vi "particle.vi"() -> ()   [LabVIEW 2017]
panel:
  in  "Strength":i32=1
  in  "Power law":i32=2
  in  "Cursor":enum16{"Attract", "Repel", "No interaction"}(ring)
  in  "Trail length":i32=500
  in  "millisecond timer value":u32=2
  in  "Drag":dbl(knob)=0.6535267495370096 scale=0.0..10.0
  in  "G":dbl[](array[numeric])=[0.0, 0.0]
  in  "Initial Velocity":dbl[](array[numeric])=[10.0, 10.0]
  in  "Initial Position":dbl[](array[numeric])=[30.0, 50.0]
  in  "?":bool
  out "XY Graph":cluster{dbl[], dbl[]}[](graph)=[{[58.5077894120906], [41.27386237710225]}, {array[500 elements], array[500 elements]}, {[46.86915887850467, 56.86915887850467, 56.86915887850467, 46.86915887850467, 46.86915887850467], [39.529262086513995, 39.529262086513995, 49.529262086513995, 49.529262086513995, 39.529262086513995]}]
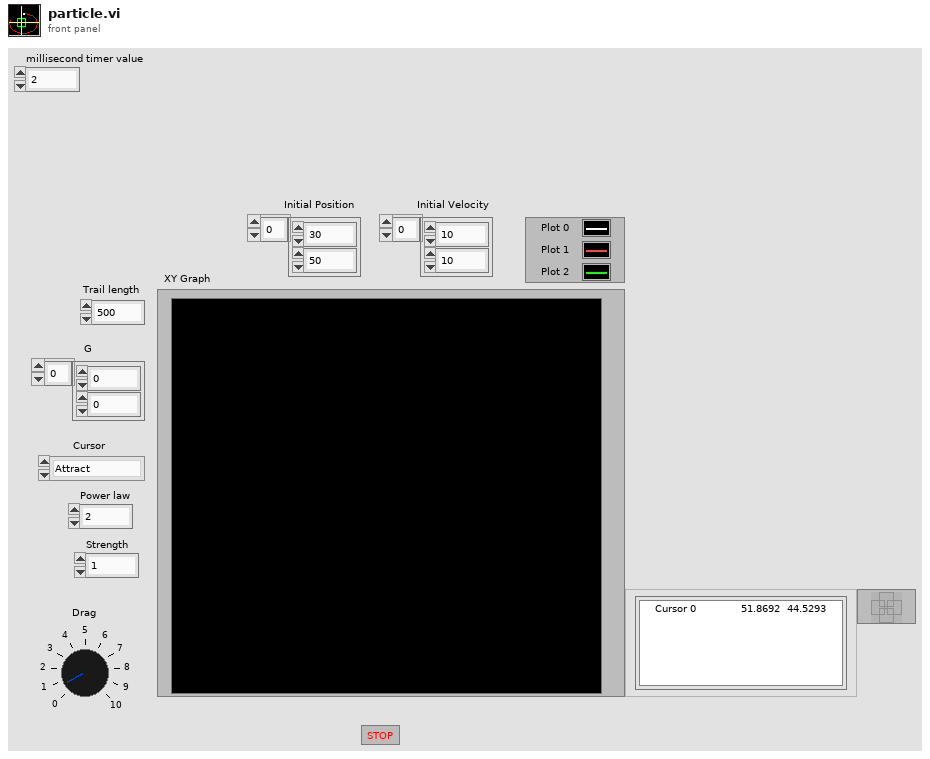
[diagram p1: front panel]
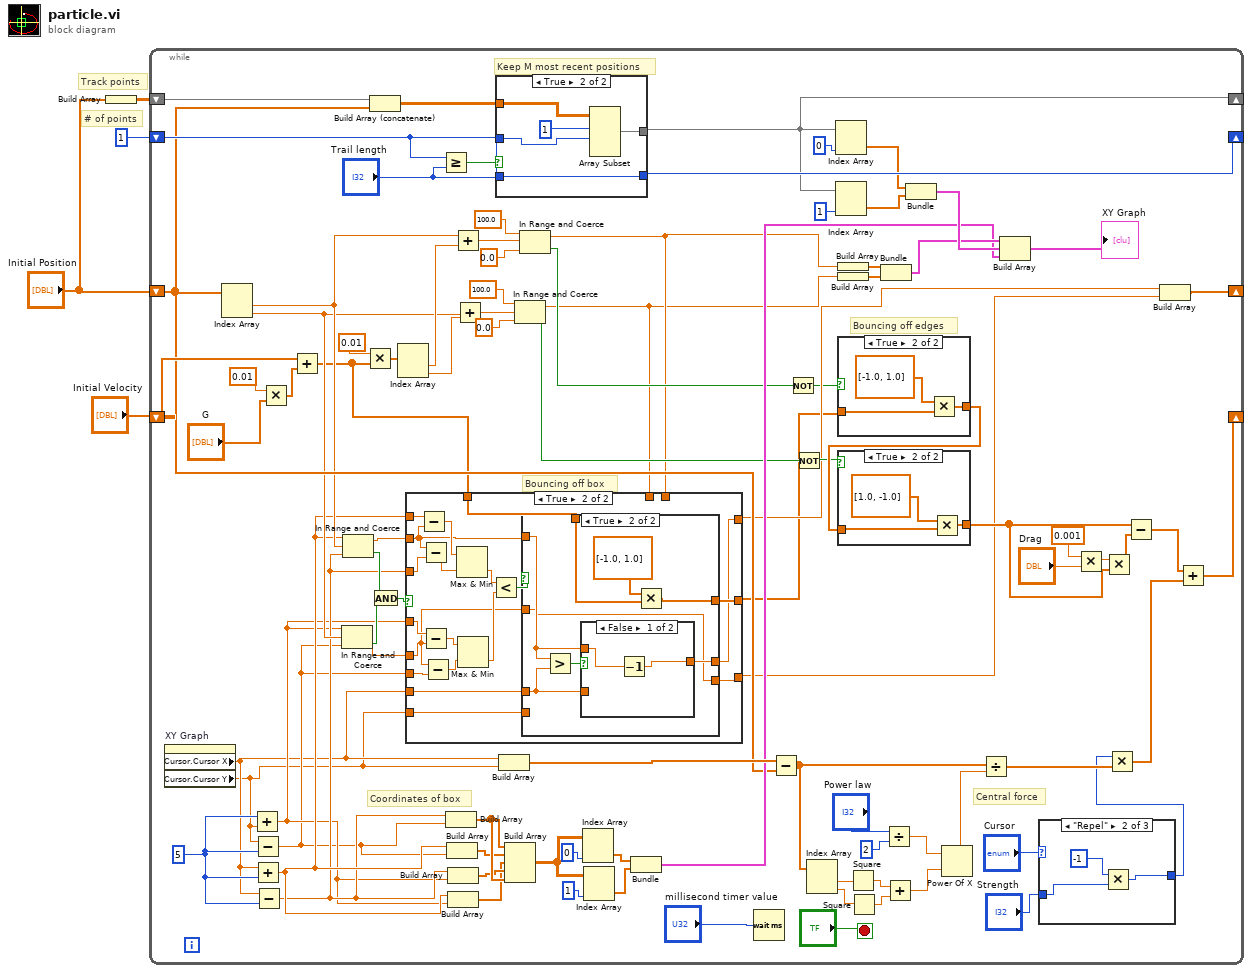
[diagram p0: block diagram]
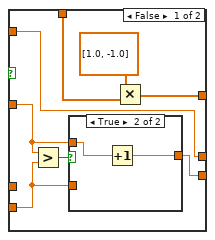
[diagram p3: hidden frame]
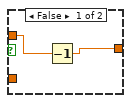
[diagram p4: hidden frame]
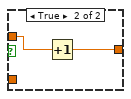
[diagram p5: hidden frame]
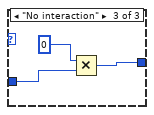
[diagram p7: hidden frame]
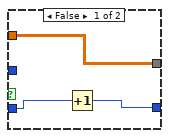
[diagram p8: hidden frame]
diagram:
  # "Track points"
  # "# of points"
  n1 = Build Array("Initial Position") -> (w3:dbl[][])
  n2 = while {
    shift-right: [w16] -> _
    shift-left: "Initial Position" -> [w32]
    shift-right: [w58] -> _
    shift-left: "Initial Velocity" -> [w79]
    shift-right: [w70] -> _
    shift-left: w3 -> [w74]
    shift-right: [w72] -> _
    shift-left: 1 -> [w68]
    stop <- "?" stop-if-true
    w42 = 5
    # "Bouncing off box"
    # "Bouncing off edges"
    # "Coordinates of box"
    # "Central force"
    # "Keep M most recent positions"
    n3 = property on="XY Graph" class="XYGraph (strict)"() -> ("Cursor.Cursor X"=w6:dbl, "Cursor.Cursor Y"=w5:dbl)  [unwired: 2 in, 2 out]
    n4 = Index Array(array=w32) -> (element #1=w30:dbl, element #2=w29:dbl)  [unwired: 2 in]
    n5 = Add(x=w42, y=w5) -> (x+y=w10:dbl)
    n6 = Subtract(x=w5, y=w42) -> (x-y=w9:dbl)
    n7 = Add(x=w6, y=w42) -> (x+y=w12:dbl)
    n8 = Subtract(x=w6, y=w42) -> (x-y=w11:dbl)
    n9 = Multiply(x=0.01, y="G") -> (x*y=w88:dbl[])
    n10 = Add(x=w79, y=w88) -> (x+y=w8:dbl[])
    n11 = In Range and Coerce(upper limit=w10, x=w29, lower limit=w9) -> (coerced(x)=w14:dbl, In Range?=w27:bool)
    n12 = In Range and Coerce(upper limit=w12, x=w30, lower limit=w11) -> (coerced(x)=w15:dbl, In Range?=w28:bool)
    n13 = Multiply(x=0.01, y=w8) -> (x*y=w84:dbl[])
    n14 = Build Array (concatenate)(w74, w32) -> (w73:dbl[][])
    n15 = And(x=w28, y=w27) -> (x .and. y?=w22:bool)
    n16 = Index Array(array=w84) -> (element #1=w81:dbl, element #2=w80:dbl)  [unwired: 2 in]
    n17 = Greater Or Equal?(x=w68, y="Trail length") -> (x >= y?=w67:bool)
    n18 = Build Array(w11, w9) -> (w35:dbl[])
    n19 = Build Array(w12, w9) -> (w31:dbl[])
    n20 = Build Array(w11, w10) -> (w34:dbl[])
    n21 = Build Array(w12, w10) -> (w33:dbl[])
    n22 = Add(x=w30, y=w81) -> (x+y=w83:dbl)
    n23 = Add(x=w29, y=w80) -> (x+y=w82:dbl)
    n24 = case shown="True" w67 {
      tunnel: w73 -> [w152 w157]
      tunnel: [w152 w155] -> w70
      tunnel: w68 -> [w151 w154]
      tunnel: [w150 w154] -> w72
      tunnel: "Trail length" -> [_ w153]
      frame False {
        n25 = Increment(x=w151) -> (x+1=w150:i32)
      }
      frame True {
        n26 = Array Subset(array=w157, index (row)=1, length (row)=w153) -> (w155:dbl[][])  [unwired: 2 in]
      }
    }
    n27 = Build Array(w6, w5) -> (w47:dbl[])
    n28 = Build Array(w35, w31, w33, w34, w35) -> (w39:dbl[][])
    n29 = In Range and Coerce(upper limit=100.0, x=w82, lower limit=0.0) -> (coerced(x)=w20:dbl, In Range?=w24:bool)
    n30 = In Range and Coerce(upper limit=100.0, x=w83, lower limit=0.0) -> (coerced(x)=w21:dbl, In Range?=w25:bool)
    n31 = case shown="True" w22 {
      tunnel: w21 -> [w99 _]
      tunnel: w20 -> [w98 _]
      tunnel: [w99 w101] -> w18
      tunnel: [w98 w100] -> w17
      tunnel: w15 -> [_ w105]
      tunnel: w14 -> [_ w104]
      tunnel: w12 -> [_ w118]
      tunnel: w11 -> [_ w117]
      tunnel: w10 -> [_ w113]
      tunnel: w9 -> [_ w112]
      tunnel: w8 -> [w97 w107]
      tunnel: [w97 w106] -> w7
      tunnel: w6 -> [_ w103]
      tunnel: w5 -> [_ w102]
      frame False {
      }
      frame True {
        n32 = Subtract(x=w118, y=w105) -> (x-y=w116:dbl)
        n33 = Subtract(x=w105, y=w117) -> (x-y=w115:dbl)
        n34 = Subtract(x=w113, y=w104) -> (x-y=w111:dbl)
        n35 = Subtract(x=w104, y=w112) -> (x-y=w114:dbl)
        n36 = Max & Min(x=w116, y=w115) -> (min(x,y)=w109:dbl)  [unwired: 1 out]
        n37 = Max & Min(x=w111, y=w114) -> (min(x,y)=w110:dbl)  [unwired: 1 out]
        n38 = Less?(x=w109, y=w110) -> (x < y?=w108:bool)
        n39 = case shown="True" w108 {
          tunnel: [w125 w137] -> w106
          tunnel: w107 -> [w124 w136]
          tunnel: w105 -> [w119 w134]
          tunnel: w104 -> [w122 w131]
          tunnel: w103 -> [_ w133]
          tunnel: w102 -> [w121 _]
          tunnel: [w119 w132] -> w101
          tunnel: [w120 w131] -> w100
          frame False {
            n40 = Greater?(x=w122, y=w121) -> (0:w123:bool)
            n41 = case shown="True" w123 {
              tunnel: w122 -> [w128 w130]
              tunnel: w121 -> [_ _]
              tunnel: [w127 w129] -> w120
              frame False {
                n42 = Decrement(x=w128) -> (x-1=w127:dbl)
              }
              frame True {
                n43 = Increment(x=w130) -> (x+1=w129:dbl)
              }
            }
            n44 = Multiply(x=dbl[] [1.0, -1.0], y=w124) -> (x*y=w125:dbl[])
          }
          frame True {
            n45 = Greater?(x=w134, y=w133) -> (0:w135:bool)
            n46 = case shown="False" w135 {
              tunnel: w134 -> [w140 w142]
              tunnel: w133 -> [_ _]
              tunnel: [w139 w141] -> w132
              frame False {
                n47 = Decrement(x=w140) -> (x-1=w139:dbl)
              }
              frame True {
                n48 = Increment(x=w142) -> (x+1=w141:dbl)
              }
            }
            n49 = Multiply(x=dbl[] [-1.0, 1.0], y=w136) -> (x*y=w137:dbl[])
          }
        }
      }
    }
    n50 = Index Array(array=w39, index (col)=0) -> (element=w38:dbl[])  [unwired: 1 in]
    n51 = Index Array(array=w39, index (col)=1) -> (element=w37:dbl[])  [unwired: 1 in]
    n52 = Bundle(w38, w37) -> (w36:cluster{dbl[], dbl[]})  [unwired: 1 in]
    n53 = Wait (ms)(milliseconds to wait="millisecond timer value") -> ()  [unwired: 1 out]
    n54 = Subtract(x=w47, y=w32) -> (x-y=w50:dbl[])
    n55 = Not(x=w25) -> (.not. x?=w13:bool)
    n56 = Not(x=w24) -> (.not. x?=w23:bool)
    n57 = Index Array(array=w50) -> (element #1=w57:dbl, element #2=w56:dbl)  [unwired: 2 in]
    n58 = Index Array(array=w70, index (col)=0) -> (element=w65:dbl[])  [unwired: 1 in]
    n59 = Index Array(array=w70, index (col)=1) -> (element=w64:dbl[])  [unwired: 1 in]
    n60 = Build Array(w21) -> (w94:dbl[])
    n61 = Build Array(w20) -> (w93:dbl[])
    n62 = case shown="True" w13 {
      tunnel: w7 -> [w162 w163]
      tunnel: [w162 w164] -> w26
      frame False {
      }
      frame True {
        n63 = Multiply(x=dbl[] [-1.0, 1.0], y=w163) -> (x*y=w164:dbl[])
      }
    }
    n64 = case shown="True" w23 {
      tunnel: w26 -> [w158 w159]
      tunnel: [w158 w160] -> w19
      frame False {
      }
      frame True {
        n65 = Multiply(x=dbl[] [1.0, -1.0], y=w159) -> (x*y=w160:dbl[])
      }
    }
    n66 = Square(x=w57) -> (x^2=w55:dbl)
    n67 = Square(x=w56) -> (x^2=w54:dbl)
    n68 = Bundle(w94, w93) -> (w62:cluster{dbl[], dbl[]})  [unwired: 1 in]
    n69 = Divide(x="Power law", y=2) -> (x/y=w51:dbl)
    n70 = Add(x=w55, y=w54) -> (x+y=w53:dbl)
    n71 = Bundle(w65, w64) -> (w63:cluster{dbl[], dbl[]})  [unwired: 1 in]
    n72 = Power Of X(1:w53, 2:w51) -> (0:w49:dbl)
    n73 = Divide(x=w50, y=w49) -> (x/y=w48:dbl[])
    n74 = Build Array(w62, w63, w36) -> (→"XY Graph":cluster{dbl[], dbl[]}[])
    n75 = case shown="\"Repel\"" "Cursor" {
      tunnel: [w143 w145 w148] -> w44
      tunnel: "Strength" -> [w143 w144 w147]
      frame "Attract", Default {
      }
      frame "Repel" {
        n76 = Multiply(x=-1, y=w144) -> (x*y=w145:i32)
      }
      frame "No interaction" {
        n77 = Multiply(x=0, y=w147) -> (x*y=w148:i32)
      }
    }
    n78 = Multiply(x=0.001, y="Drag") -> (x*y=w76:dbl)
    n79 = Multiply(x=w76, y=w19) -> (x*y=w78:dbl[])
    n80 = Multiply(x=w44, y=w48) -> (x*y=w46:dbl[])
    n81 = Subtract(x=w19, y=w78) -> (x-y=w59:dbl[])
    n82 = Build Array(w18, w17) -> (w16:dbl[])
    n83 = Add(x=w59, y=w46) -> (x+y=w58:dbl[])
  }
